vi "copy.vi"(8 "error in (no error)":errorcluster, 10 "ScriptEventForCopy":refnum<class "ScriptEvent.lvclass">, 11 "RfRamp in":refnum<class "RfRamp.lvclass">) -> (0 "error out":errorcluster, 3 "RfRamp out":refnum<class "RfRamp.lvclass">)   [LabVIEW 2011, in "Tools.lvlib" / "Scripting.lvlib" / "RfRamp.lvclass"]
uses:
  RfRamp.lvclass
  ScriptEvent.lvclass
  RfRamp.lvclass/RfRamp.ctl
  Rf Event/rf.lvclass
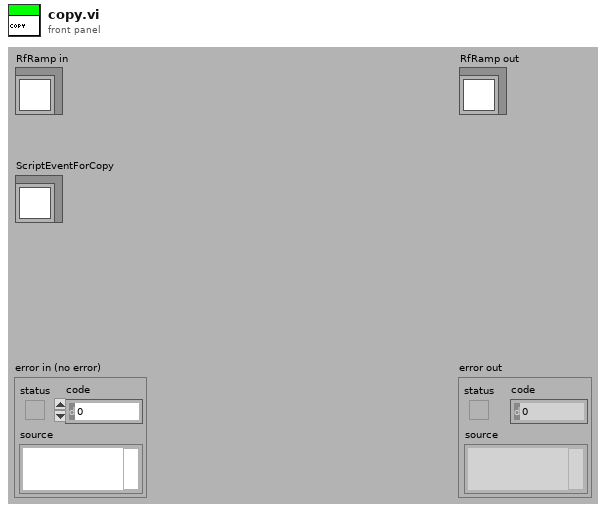
[diagram p1: front panel]
types:
  T1 = enum16{"changeValue", "pulse", "clock", "rampUp", "rampDown", "singleTone", "singleToneRamp", "playFile", "rf", "rfRamp", "delay"}
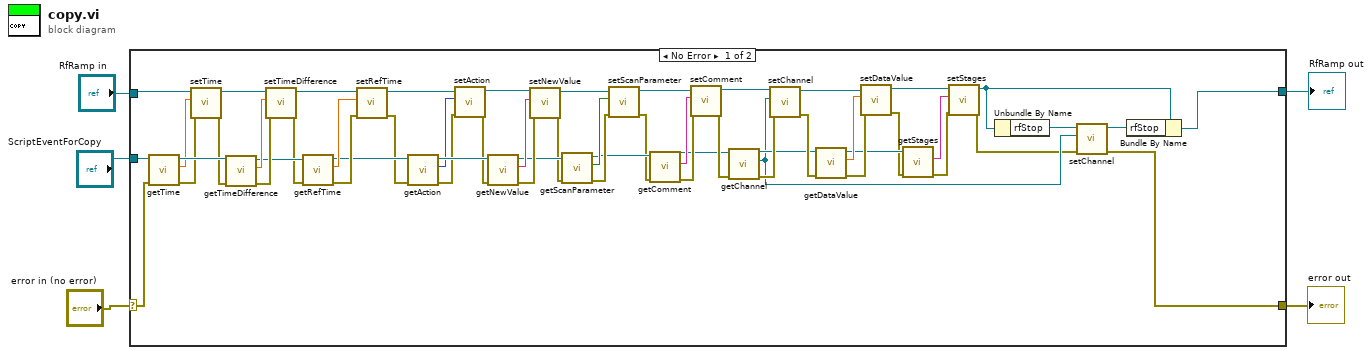
[diagram p0: block diagram]
diagram:
  n1 = case shown="No Error" "error in (no error)" {
    selector: "error in (no error)" -> [w15 w62]
    tunnel: [w7 w63] -> w4
    tunnel: "RfRamp in" -> [w16 w63]
    tunnel: [w8 w62] -> w2
    tunnel: "ScriptEventForCopy" -> [w14 _]
    frame No Error {
      n2 = call "getTime.vi"("error in (no error)"=w15, "ScriptEvent.lvclass in"=w14) -> ("error out"=w60:errorcluster, "time"=w59:dbl, "ScriptEvent.lvclass out"=w61:refnum<class "ScriptEvent.lvclass">)  [unwired: 7 in]
      n3 = call "setTime.vi"("error in (no error)"=w60, "time"=w59, "ScriptEvent.lvclass in"=w16) -> ("error out"=w58:errorcluster, "ScriptEvent.lvclass out"=w31:refnum<class "RfRamp.lvclass">)  [unwired: 7 in]
      n4 = call "getTimeDifference.vi"("error in (no error)"=w58, "ScriptEvent.lvclass in"=w61) -> ("error out"=w57:errorcluster, "time difference"=w32:dbl, "ScriptEvent.lvclass out"=w22:refnum<class "ScriptEvent.lvclass">)  [unwired: 7 in]
      n5 = call "setTimeDifference.vi"("error in (no error)"=w57, "time difference"=w32, "ScriptEvent.lvclass in"=w31) -> ("error out"=w21:errorcluster, "ScriptEvent.lvclass out"=w23:refnum<class "RfRamp.lvclass">)  [unwired: 7 in]
      n6 = call "getRefTime.vi"("error in (no error)"=w21, "ScriptEvent.lvclass in"=w22) -> ("error out"=w19:errorcluster, "refTime"=w20:dbl, "ScriptEvent.lvclass out"=w18:refnum<class "ScriptEvent.lvclass">)  [unwired: 7 in]
      n7 = call "setRefTime.vi"("error in (no error)"=w19, "refTime"=w20, "ScriptEvent.lvclass in"=w23) -> ("error out"=w17:errorcluster, "ScriptEvent.lvclass out"=w24:refnum<class "RfRamp.lvclass">)  [unwired: 7 in]
      n8 = call "getAction.vi"("error in (no error)"=w17, "ScriptEvent.lvclass in"=w18) -> ("error out"=w55:errorcluster, "action"=w54:T1, "ScriptEvent.lvclass out"=w56:refnum<class "ScriptEvent.lvclass">)  [unwired: 7 in]
      n9 = call "setAction.vi"("error in (no error)"=w55, "action"=w54, "ScriptEvent.lvclass in"=w24) -> ("error out"=w53:errorcluster, "ScriptEvent.lvclass out"=w30:refnum<class "RfRamp.lvclass">)  [unwired: 7 in]
      n10 = call "getNewValue.vi"("error in (no error)"=w53, "ScriptEvent.lvclass in"=w56) -> ("error out"=w52:errorcluster, "newValue"=w51:string, "ScriptEvent.lvclass out"=w50:refnum<class "ScriptEvent.lvclass">)  [unwired: 7 in]
      n11 = call "setNewValue.vi"("error in (no error)"=w52, "newValue"=w51, "ScriptEvent.lvclass in"=w30) -> ("error out"=w49:errorcluster, "ScriptEvent.lvclass out"=w29:refnum<class "RfRamp.lvclass">)  [unwired: 7 in]
      n12 = call "getScanParameter.vi"("error in (no error)"=w49, "ScriptEvent.lvclass in"=w50) -> ("error out"=w47:errorcluster, "scanParameter"=w48:bool, "ScriptEvent.lvclass out"=w46:refnum<class "ScriptEvent.lvclass">)  [unwired: 7 in]
      n13 = call "setScanParameter.vi"("error in (no error)"=w47, "scanParameter"=w48, "ScriptEvent.lvclass in"=w29) -> ("error out"=w45:errorcluster, "ScriptEvent.lvclass out"=w28:refnum<class "RfRamp.lvclass">)  [unwired: 7 in]
      n14 = call "getComment.vi"("error in (no error)"=w45, "ScriptEvent.lvclass in"=w46) -> ("error out"=w44:errorcluster, "comment"=w43:string, "ScriptEvent.lvclass out"=w41:refnum<class "ScriptEvent.lvclass">)  [unwired: 7 in]
      n15 = call-dynamic "setComment.vi"("error in (no error)"=w44, "comment"=w43, "RfRamp.lvclass in"=w28) -> ("error out"=w42:errorcluster, "RfRamp.lvclass out"=w27:refnum<class "RfRamp.lvclass">)  [unwired: 7 in]
      n16 = call-dynamic "getChannel.vi"("error in (no error)"=w42, "ScriptEvent.lvclass in"=w41) -> ("error out"=w40:errorcluster, "Channel.lvclass"=w12:refnum<class "Channel.lvclass">, "ScriptEvent.lvclass out"=w38:refnum<class "ScriptEvent.lvclass">)  [unwired: 7 in]
      n17 = call-dynamic "setChannel.vi"("error in (no error)"=w40, "Channel.lvclass"=w12, "RfRamp.lvclass in"=w27) -> ("error out"=w39:errorcluster, "RfRamp.lvclass out"=w26:refnum<class "RfRamp.lvclass">)  [unwired: 7 in]
      n18 = call "getDataValue.vi"("error in (no error)"=w39, "ScriptEvent.lvclass in"=w38) -> ("error out"=w37:errorcluster, "dataValue"=w36:dbl, "ScriptEvent.lvclass out"=w35:refnum<class "ScriptEvent.lvclass">)  [unwired: 7 in]
      n19 = call "setDataValue.vi"("error in (no error)"=w37, "dataValue"=w36, "ScriptEvent.lvclass in"=w26) -> ("error out"=w34:errorcluster, "ScriptEvent.lvclass out"=w25:refnum<class "RfRamp.lvclass">)  [unwired: 7 in]
      n20 = call "getStages.vi"("error in (no error)"=w34, "ScriptEvent.lvclass in"=w35) -> ("error out"=w6:errorcluster, "Stage"=w33:string)  [unwired: 7 in, 1 out]
      n21 = call-dynamic "setStages.vi"("error in (no error)"=w6, "Stage"=w33, "RfRamp.lvclass in"=w25) -> ("error out"=w11:errorcluster, "RfRamp.lvclass out"=w10:refnum<class "RfRamp.lvclass">)  [unwired: 7 in]
      n22 = Unbundle By Name(w10) -> ("rfStop"=w13:refnum<class "rf.lvclass">)
      n23 = call-dynamic "setChannel.vi"("error in (no error)"=w11, "Channel.lvclass"=w12, "rf.lvclass in"=w13) -> ("error out"=w8:errorcluster, "rf.lvclass out"=w9:refnum<class "rf.lvclass">)  [unwired: 7 in]
      n24 = Bundle By Name(cluster=w10, "rfStop"=w9) -> (w7:refnum<class "RfRamp.lvclass">)
    }
    frame Error {
    }
  }
  "error out" <- w2
  "RfRamp out" <- w4
